vi "macro_BoolCmd_Send.vi"   [LabVIEW 2019, in "Trajectory_Library.lvlib"]
uses:
  VI/DigSeqLogic_Edge_On.vi
  VI/BoolCmd_Send_Internal.vi
  VI/BoolCmd_ObtainQueue.vi
  Trajectory_Library.lvlib
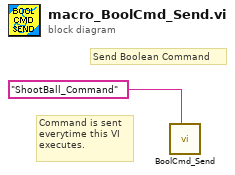
[diagram p0: block diagram]
diagram:
  # "Command is sent\neverytime this VI\nexecutes."
  # "Send Boolean Command"
  n1 = call "BoolCmd_Send.vi"("Command Name"="ShootBall_Command") -> ()  [unwired: 10 in, 1 out]
